vi "MockDigitalOutput.vi"(11 "MockDigitalOutput":cluster{"BufferUpdateFIFO":refnum<k21>}={"BufferUpdateFIFO"="MockDigitalOutputCommand"}) -> ()   [LabVIEW 2016, in "FPGAMockDigitalOutput.lvlib"]
uses:
  FPGAMockDigitalOutput.lvlib
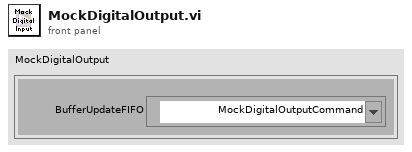
[diagram p1: front panel]
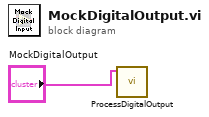
[diagram p0: block diagram]
diagram:
  n1 = call "ProcessDigitalOutput.vi"("MockDigitalOutput"="MockDigitalOutput") -> ()  [unwired: 11 in]
